vi "Position RTH Button Underneath.vi"(8 "error in (no error)":errorcluster, 10 "Previous Button":refnum<vi>, 11 "Fly Button Ref":refnum<vi>) -> (0 "error out":errorcluster)   [LabVIEW 2014]
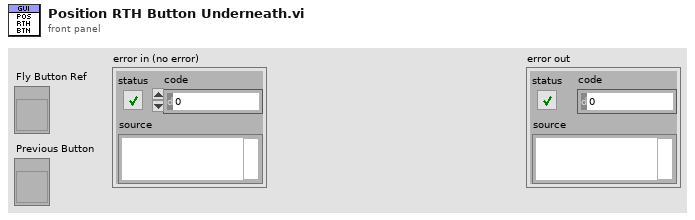
[diagram p1: front panel]
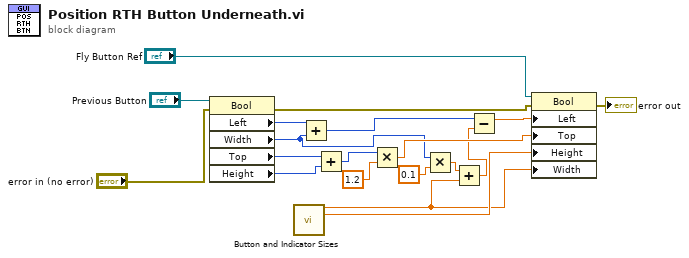
[diagram p0: block diagram]
diagram:
  n1 = property class="Bool"(reference="Previous Button", error in="error in (no error)") -> (error out=w18:errorcluster, "Left"=w11:i32, "Width"=w5:u32, "Top"=w12:i32, "Height"=w14:u32)  [unwired: 1 out]
  n2 = call "Button and Indicator Sizes.vi"() -> ("Button Width"=w2:dbl, "Button Height"=w13:dbl)  [unwired: 11 in, 3 out]
  n3 = Add(x=w11, y=w5) -> (x+y=w10:u32)
  n4 = Add(x=w12, y=w14) -> (x+y=w8:u32)
  n5 = Multiply(x=w8, y=1.2) -> (x*y=w6:dbl)
  n6 = Multiply(x=w5, y=0.1) -> (x*y=w3:dbl)
  n7 = Add(x=w3, y=w2) -> (x+y=w1:dbl)
  n8 = Subtract(x=w10, y=w1) -> (x-y=w9:dbl)
  n9 = property class="Bool"(reference="Fly Button Ref", error in=w18, "Left"=w9, "Top"=w6, "Height"=w13, "Width"=w2) -> (error out=→"error out":errorcluster)  [unwired: 1 out]
